vi "test Add Label Error.vi"(8 "error in":errorcluster, 11 "TestCase in":refnum<class "Scripting.lvclass">) -> (0 "error out":errorcluster, 3 "TestCase out":refnum<class "Scripting.lvclass">)   [LabVIEW 2020, in "Scripting.lvclass"]
uses:
  Scripting.lvclass
  <vilib>/addons/_JKI Toolkits/VI Tester/TestCase.llb/TestCase.lvclass
  Scripting/Ballard/Ballard ARINC 429 Scripting.lvlib
  Shared/Direction.ctl
  Shared/SDI.ctl
  Shared/Transfer Type.ctl
  Shared/Transfer Speed.ctl
  C:/Program Files (x86)/National Instruments/LabVIEW 2020/vi.lib/addons/_JKI Toolkits/VI Tester/TestCase.llb/TestCase.lvclass
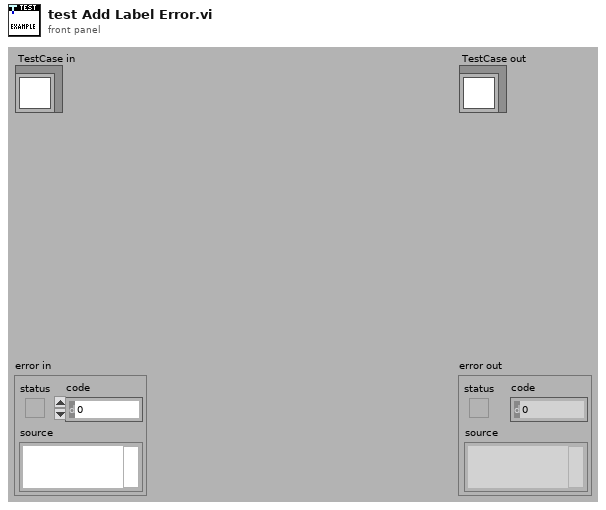
[diagram p1: front panel]
types:
  T1 = typedef "Transfer Speed.ctl" = enum16{"LO (12.5 kb/s)", "HI (100 kb/s)"}
  T2 = typedef "Transfer Type.ctl" = enum16{"Scheduled", "Acyclic", "Block", "Strobe"}
  T3 = typedef "Direction.ctl" = enum16{"Rx", "Tx"}
  T4 = cluster{"SDI":bool, "SSM":bool, "Parity":bool, "Timestamp":bool}
  T5 = typedef "SDI.ctl" = i32
  T6 = typedef "Custom Device API.lvlib/Custom Device Item Ref.ctl" = u64
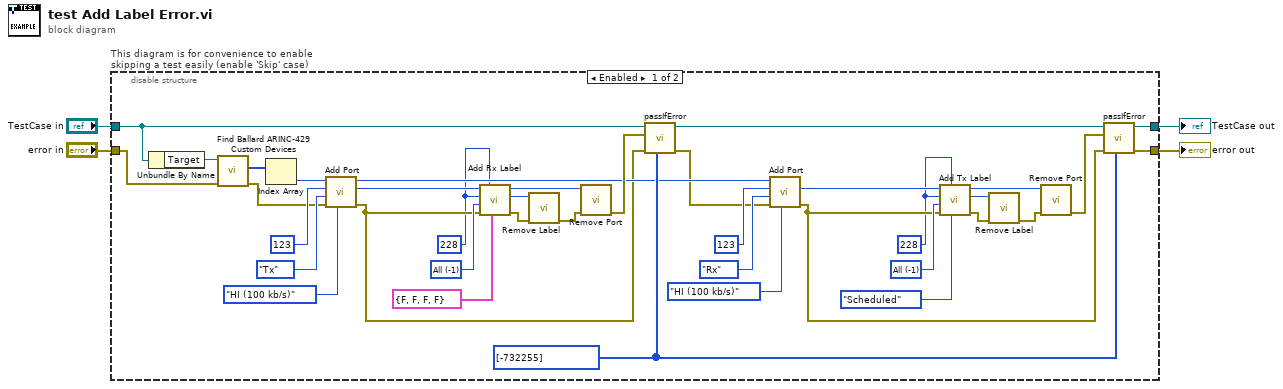
[diagram p0: block diagram]
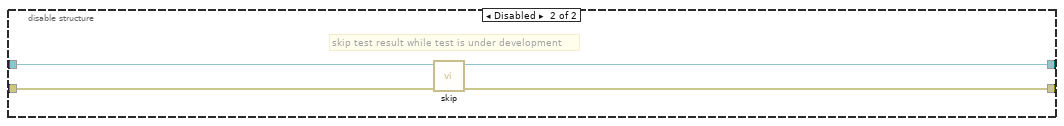
[diagram p2: hidden frame]
diagram:
  n1 = disable-structure "This diagram is for convenience to enable skipping a test easily (enable 'Skip' case)" shown="Enabled" {
    disable-tunnel: "TestCase in" -> [w39 w46]
    disable-tunnel: [w10 w44] -> w1
    disable-tunnel: [w9 w45] -> w3
    disable-tunnel: "error in" -> [w41 w43]
    frame Enabled {
      w6 = u32 228 ("label value")
      w23 = T5 -1 items=["All"=-1, "0 (b00)"=0, "1 (b01)"=1, "2 (b10)"=2, "3 (b11)"=3] ("SDI value")
      w17 = i32[] [-732255] ("passing error codes (default = any error code)")
      w5 = u32 228 ("label value")
      w37 = T5 -1 items=["All"=-1, "0 (b00)"=0, "1 (b01)"=1, "2 (b10)"=2, "3 (b11)"=3] ("SDI value")
      n2 = Unbundle By Name(w39) -> ("Target"=w42:refnum<k24>)
      n3 = call "Find Ballard ARINC-429 Custom Devices.vi"("error in"=w41, "target in"=w42) -> ("error out"=w19:errorcluster, "Ballard ARINC 429 custom devices"=w40:u64[])  [unwired: 7 in, 1 out]
      n4 = Index Array(array=w40) -> (element=w36:u64)  [unwired: 1 in]
      n5 = call "Add Port.vi"("speed (HI 100 kb/s)"=Transfer_Speed."HI (100 kb/s)" ("speed"), "error in"=w19, "direction"=Direction."Tx", "port number"=u16 123, "Ballard ARINC 429 custom device in"=w36) -> ("error out"=w13:errorcluster, "port"=w33:T6, "Ballard ARINC 429 custom device out"=w14:T6)  [unwired: 4 in]
      n6 = call "Add Rx Label.vi"("create channels"=T4 {"SDI"=FALSE, "SSM"=FALSE, "Parity"=FALSE, "Timestamp"=FALSE}, "label (Dec or Oct)"=w5, "error in"=w13, "SDI value"=w37, "label (Dec)"=w5, "port in"=w33) -> ("error out"=w18:errorcluster, "label"=w30:T6, "port out"=w38:T6)  [unwired: 3 in]
      n7 = call "Remove Label.vi"("error in"=w18, "label"=w30) -> ("error out"=w32:errorcluster)  [unwired: 9 in]
      n8 = call "Remove Port.vi"("error in"=w32, "port"=w38) -> ("error out"=w15:errorcluster)  [unwired: 9 in]
      n9 = call-dynamic "passIfError.vi"("passing error codes (default = any error code)"=w17, "error in (no error)"=w13, "error"=w15, "TestCase in"=w39) -> ("error out"=w12:errorcluster, "TestCase out"=w20:refnum<class "Scripting.lvclass">)  [unwired: 6 in]
      n10 = call "Add Port.vi"("speed (HI 100 kb/s)"=Transfer_Speed."HI (100 kb/s)" ("speed"), "error in"=w12, "direction"=Direction."Rx", "port number"=u16 123, "Ballard ARINC 429 custom device in"=w14) -> ("error out"=w11:errorcluster, "port"=w26:T6)  [unwired: 4 in, 1 out]
      n11 = call "Add Tx Label.vi"("transfer type"=Transfer_Type."Scheduled", "label (Dec or Oct)"=w6, "error in"=w11, "SDI value"=w23, "label (Dec)"=w6, "port in"=w26) -> ("error out"=w28:errorcluster, "label"=w29:T6, "port out"=w22:T6)  [unwired: 3 in]
      n12 = call "Remove Label.vi"("error in"=w28, "label"=w29) -> ("error out"=w27:errorcluster)  [unwired: 9 in]
      n13 = call "Remove Port.vi"("error in"=w27, "port"=w22) -> ("error out"=w16:errorcluster)  [unwired: 9 in]
      n14 = call-dynamic "passIfError.vi"("passing error codes (default = any error code)"=w17, "error in (no error)"=w11, "error"=w16, "TestCase in"=w20) -> ("error out"=w9:errorcluster, "TestCase out"=w10:refnum<class "Scripting.lvclass">)  [unwired: 6 in]
    }
    frame Disabled {
      # "skip test result while test is under development"
      n15 = call <vilib>:"skip.vi"("error in (no error)"=w43, "TestCase in"=w46) -> ("error out"=w45:errorcluster, "TestCase out"=w44:refnum<class "Scripting.lvclass">)  [unwired: 8 in]
    }
  }
  "error out" <- w3
  "TestCase out" <- w1
